vi "LDO Trigger Events.vi"(0 "Event Booleans in":T1, 1 "Burner ON Ref":refnum<vi>, 2 "0.8 ML Ref":refnum<vi>, 3 "1.1 ML Ref":refnum<vi>, 4 "1.33 ML Ref":refnum<vi>, 5 "error in":errorcluster, 6 "Start recording data":refnum<vi>, 7 "Oil spray 0.8cc/min - LDO":bool, 8 "Burner ON":bool, 9 "Oil spray 1.1cc/min - LDO":bool, 11 "Oil spray 1.33cc/min - LDO":bool, 13 "Start recording data-LDO":bool) -> (14 "Event Booleans out":T1, 19 "error out":errorcluster)   [LabVIEW 2020]
uses:
  Event Booleans.ctl
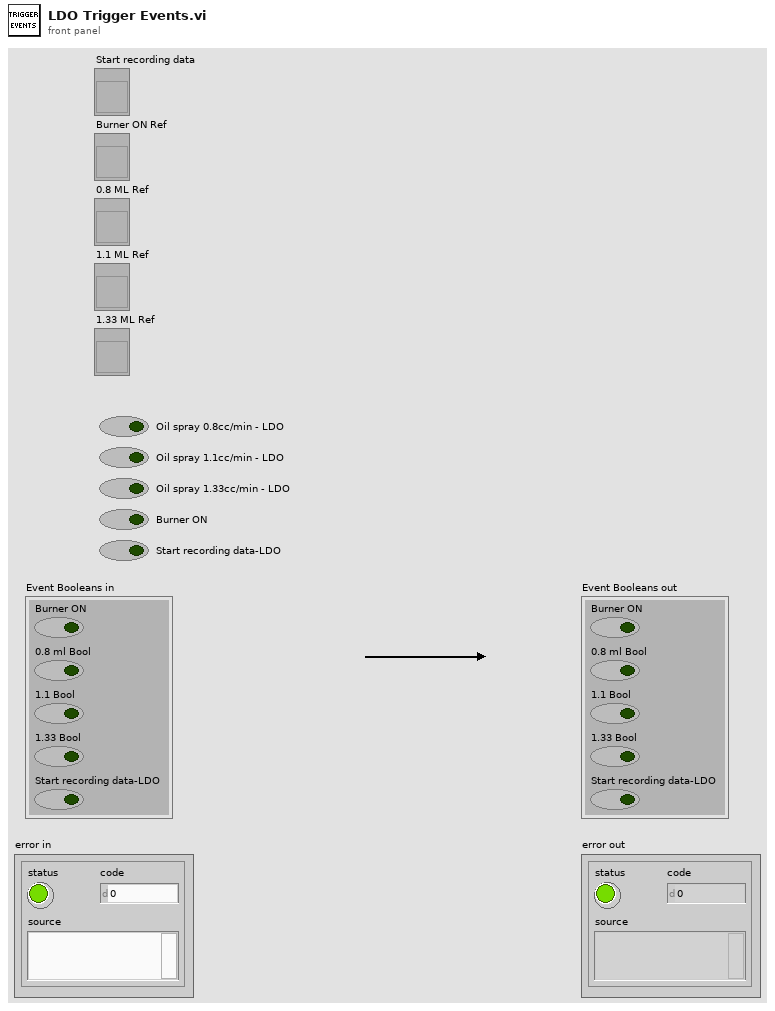
[diagram p1: front panel]
types:
  T1 = typedef "Event Booleans.ctl" = cluster{"Burner ON":bool, "0.8 ml Bool":bool, "1.1 Bool":bool, "1.33 Bool":bool, "Start recording data-LDO":bool}
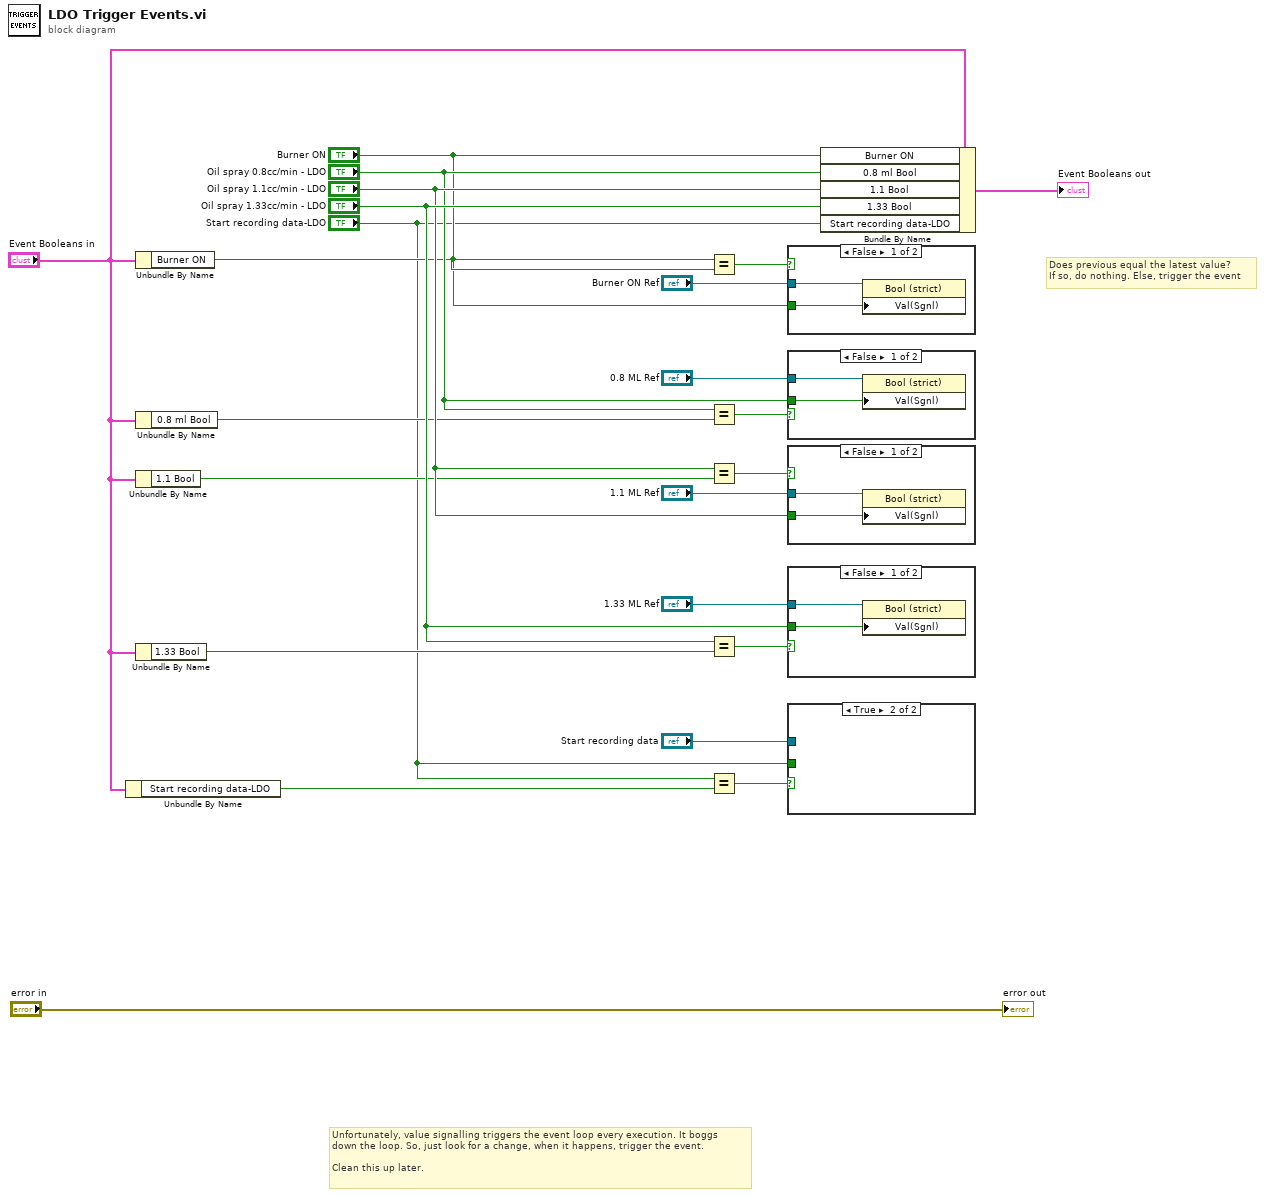
[diagram p0: block diagram]
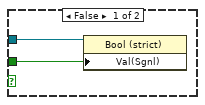
[diagram p2: hidden frame]
diagram:
  # "Does previous equal the latest value?\nIf so, do nothing. Else, trigger the event"
  # "Unfortunately, value signalling triggers the event loop every execution. It boggs\ndown the loop. So, just look for a change, when it happens, trigger the event. \n\nClean this up later."
  n1 = Unbundle By Name("Event Booleans in") -> ("Start recording data-LDO"=w2:bool)
  n2 = Unbundle By Name("Event Booleans in") -> ("Burner ON"=w11:bool)
  n3 = Unbundle By Name("Event Booleans in") -> ("0.8 ml Bool"=w10:bool)
  n4 = Unbundle By Name("Event Booleans in") -> ("1.1 Bool"=w9:bool)
  n5 = Unbundle By Name("Event Booleans in") -> ("1.33 Bool"=w8:bool)
  n6 = Equal?(x="Burner ON", y=w11) -> (x = y?=w16:bool)
  n7 = Equal?(x="Oil spray 0.8cc/min - LDO", y=w10) -> (x = y?=w18:bool)
  n8 = Equal?(x="Oil spray 1.1cc/min - LDO", y=w9) -> (x = y?=w20:bool)
  n9 = Equal?(x="Oil spray 1.33cc/min - LDO", y=w8) -> (x = y?=w19:bool)
  n10 = Equal?(x="Start recording data-LDO", y=w2) -> (x = y?=w5:bool)
  n11 = case shown="False" w16 {
    tunnel: "Burner ON" -> [w25 _]
    tunnel: "Burner ON Ref" -> [w24 _]
    frame False {
      n12 = property on="Property Node" class="Bool (strict)"(reference=w24, "Val(Sgnl)"=w25) -> ()  [unwired: 1 in, 2 out]
    }
    frame True {
    }
  }
  n13 = case shown="False" w18 {
    tunnel: "Oil spray 0.8cc/min - LDO" -> [w27 _]
    tunnel: "0.8 ML Ref" -> [w26 _]
    frame False {
      n14 = property on="Property Node" class="Bool (strict)"(reference=w26, "Val(Sgnl)"=w27) -> ()  [unwired: 1 in, 2 out]
    }
    frame True {
    }
  }
  n15 = case shown="False" w20 {
    tunnel: "Oil spray 1.1cc/min - LDO" -> [w29 _]
    tunnel: "1.1 ML Ref" -> [w28 _]
    frame False {
      n16 = property on="Property Node" class="Bool (strict)"(reference=w28, "Val(Sgnl)"=w29) -> ()  [unwired: 1 in, 2 out]
    }
    frame True {
    }
  }
  n17 = case shown="False" w19 {
    tunnel: "Oil spray 1.33cc/min - LDO" -> [w31 _]
    tunnel: "1.33 ML Ref" -> [w30 _]
    frame False {
      n18 = property on="Property Node" class="Bool (strict)"(reference=w30, "Val(Sgnl)"=w31) -> ()  [unwired: 1 in, 2 out]
    }
    frame True {
    }
  }
  n19 = case shown="True" w5 {
    tunnel: "Start recording data-LDO" -> [w32 _]
    tunnel: "Start recording data" -> [w33 _]
    frame False {
      n20 = property on="Property Node" class="Bool (strict)"(reference=w33, "Val(Sgnl)"=w32) -> ()  [unwired: 1 in, 2 out]
    }
    frame True {
    }
  }
  n21 = Bundle By Name(cluster="Event Booleans in", "Burner ON"="Burner ON", "0.8 ml Bool"="Oil spray 0.8cc/min - LDO", "1.1 Bool"="Oil spray 1.1cc/min - LDO", "1.33 Bool"="Oil spray 1.33cc/min - LDO", "Start recording data-LDO"="Start recording data-LDO") -> (→"Event Booleans out":T1)
  "error out" <- "error in"
